vi "read_waveform.vi"(8 "error in (no error)":errorcluster, 10 "Small?":bool, 11 "Dust Event ID":i32) -> (0 "error out":errorcluster, 2 "multiplier":dbl, 3 "Waveform":T1)   [LabVIEW 2013]
uses:
  User Interface/Controls/Waveforms.ctl
  <vilib>/addons/h5labview/H5F_mode.ctl
  User Interface/Controls/Post_Signal.ctl
  User Interface/Controls/Role ID.ctl
  User Interface/Controls/Hardware ID.ctl
  <userlib>/_OpenG.lib/file/file.llb/File Exists - Scalar__ogtk.vi
  <vilib>/addons/h5labview/polymorph/H5A_read_var.vi
  <vilib>/addons/database/_DB Variant To Data/Database Variant To Data.xnode
  <vilib>/addons/h5labview/H5File.lvlib
  <vilib>/addons/h5labview/H5GroupObject.lvlib
  <vilib>/addons/h5labview/H5Attrib.lvlib
panel:
  out "Query Syntax":string
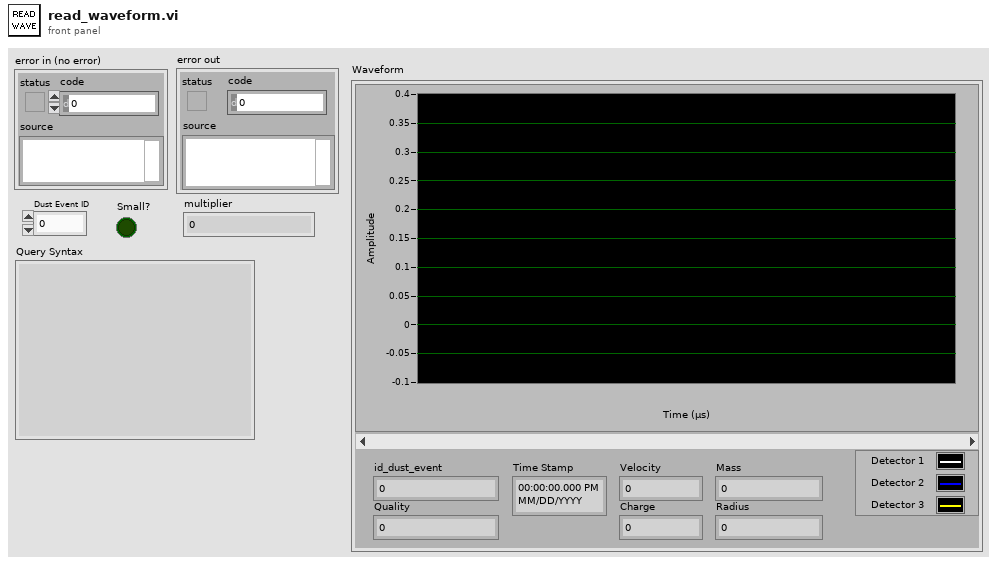
[diagram p1: front panel]
types:
  T1 = typedef "Waveforms.ctl" = cluster{"id_dust_event":u64, "Time Stamp":timestamp, "Velocity":dbl, "Mass":dbl, "Charge":dbl, "Radius":dbl, "Waveform Graph":sgl[][], "Quality":i32}
  T2 = typedef "H5File.lvlib/H5F_mode.ctl" = enum16{"read-only", "read-write", "overwrite", "create new", "open or create"}
  T3 = typedef "Role ID.ctl" = enum16{"First_Detector", "Second_Detector", "Third_Detector", "LeCroy_CH1", "LeCroy_CH2", "LeCroy_CH3", "LeCroy_CH4", "PSU", "DCS 1", "DCS 2"}
  T4 = typedef "Post_Signal.ctl" = cluster{"Integer Timestamp":i64, "Dust Event ID":i64, "Role ID":T3, "Data":sgl[], "Signal Length":i32, "dt":sgl, "Offset":dbl, "Hardware ID":T5}
  T5 = typedef "Hardware ID.ctl" = enum16{"Unknown", "CSA 1", "CSA 2", "CSA 3", "CSA 4", "CSA 5", "CSA 6", "DCS 1", "DCS 2"}
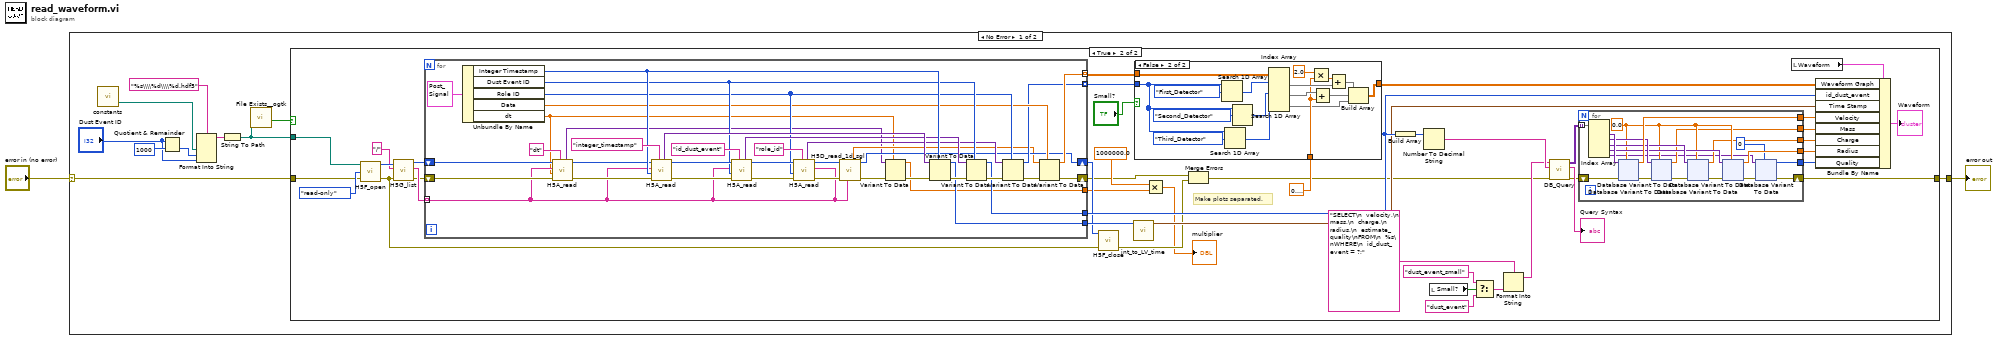
[diagram p0: block diagram]
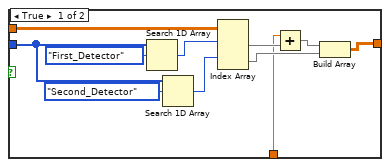
[diagram p3: hidden frame]
diagram:
  n1 = case shown="No Error" "error in (no error)" {
    selector: "error in (no error)" -> [w3 w302]
    tunnel: [w7 w302] -> w1
    frame No Error {
      n2 = call "constants.vi"() -> ("file path for Processed Signal .hdf5 files"=w4:path)  [unwired: 3 in, 2 out]
      n3 = Quotient & Remainder(x="Dust Event ID", y=1000) -> (floor(x/y)=w10:i32)  [unwired: 1 out]
      n4 = Format Into String(format string="%s\\\\%d\\\\%d.hdf5", w4, w10, "Dust Event ID") -> (resulting string=w8:string)  [unwired: 2 in, 1 out]
      n5 = String To Path(string=w8) -> (path=w5:path)
      n6 = call-poly <userlib>:"File Exists__ogtk.vi"("file path"=w5) -> ("exists"=w6:bool)  [unwired: 6 in, 1 out]
      n7 = case shown="True" w6 {
        tunnel: w5 -> [_ w56]
        tunnel: [w13 w54] -> w7
        tunnel: w3 -> [w13 w14]
        frame False {
        }
        frame True {
          # "Make plots separated."
          n8 = call <vilib>:"H5F_open.vi"("error in (no error)"=w14, "mode"=H5F_mode."read-only", "path"=w56) -> ("error out"=w20:errorcluster, "ref"=w53:i32)  [unwired: 1 in]
          n9 = call <vilib>:"H5G_list.vi"("error in (no error)"=w20, "group"="/", "ref"=w53) -> ("error out"=w25:errorcluster, "names"=w29:string[], "ref out"=w26:i32)  [unwired: 1 in, 1 out]
          n10 = for {
            shift-right: [w279] -> w17
            shift-left: w25 -> [w272]
            shift-right: [w278] -> w27
            shift-left: w26 -> [w274]
            tunnel: w29 -> [w265] mode=indexing
            tunnel: [w280] -> w31 mode=indexing
            tunnel: [w281] -> w32 mode=indexing
            tunnel: [w276] -> w50
            tunnel: [w277] -> w33
            tunnel: [w267] -> w15
            n11 = Unbundle By Name(T4 {"Integer Timestamp"=0, "Dust Event ID"=0, "Role ID"=enum."First_Detector", "Data"=[], "Signal Length"=0, "dt"=0.0, "Offset"=0.0, "Hardware ID"=enum."CSA 1"} ("Post_Signal 2")) -> ("Integer Timestamp"=w299:i64, "Dust Event ID"=w293:i64, "Role ID"=w287:T3, "Data"=w284:sgl[], "dt"=w264:sgl)
            n12 = call-poly <vilib>:"H5A_read.vi"("attrib_name"="dt", "error in (no error)"=w272, "default"=w264, "obj_name"=w265, "ref"=w274) -> ("error out"=w271:errorcluster, "ref out"=w273:i32, "value"=w268:variant)  [unwired: 2 in]
            n13 = call-poly <vilib>:"H5A_read.vi"("attrib_name"="integer_timestamp", "error in (no error)"=w271, "default"=w299, "obj_name"=w265, "ref"=w273) -> ("error out"=w295:errorcluster, "ref out"=w297:i32, "value"=w298:variant)  [unwired: 2 in]
            n14 = call-poly <vilib>:"H5A_read.vi"("attrib_name"="id_dust_event", "error in (no error)"=w295, "default"=w293, "obj_name"=w265, "ref"=w297) -> ("error out"=w291:errorcluster, "ref out"=w290:i32, "value"=w294:variant)  [unwired: 2 in]
            n15 = call-poly <vilib>:"H5A_read.vi"("attrib_name"="role_id", "error in (no error)"=w291, "default"=w287, "obj_name"=w265, "ref"=w290) -> ("error out"=w282:errorcluster, "ref out"=w283:i32, "value"=w288:variant)  [unwired: 2 in]
            n16 = call "H5D_read_1d_sgl.vi"("name"=w265, "error in (no error)"=w282, "ref"=w283) -> ("error out"=w270:errorcluster, "ref out"=w278:i32, "data"=w275:sgl[])  [unwired: 4 in]
            n17 = Variant To Data(error in=w270, type=w264, Variant=w268) -> (data=w267:sgl, error out=w269:errorcluster)
            n18 = Variant To Data(error in=w269, type=w299, Variant=w298) -> (data=w277:i64, error out=w292:errorcluster)
            n19 = Variant To Data(error in=w292, type=w293, Variant=w294) -> (data=w276:i64, error out=w286:errorcluster)
            n20 = Variant To Data(error in=w286, type=w287, Variant=w288) -> (data=w280:T3, error out=w285:errorcluster)
            n21 = Variant To Data(error in=w285, type=w284, Variant=w275) -> (data=w281:sgl[], error out=w279:errorcluster)
          }
          n22 = call <vilib>:"H5F_close.vi"("error in (no error)"=w20, "ref"=w27) -> ("error out"=w21:errorcluster)  [unwired: 3 in]
          n23 = call "int_to_LV_time.vi"("Integer Timestamp"=w33) -> ("time stamp"=w34:timestamp)  [unwired: 8 in, 1 out]
          n24 = case shown="False" "Small?" {
            tunnel: w31 -> [w243 w259]
            tunnel: w32 -> [w241 w256]
            tunnel: [w238 w251] -> w23
            tunnel: sgl 0.1 -> [w236 w248]
            frame True {
              n25 = Search 1D Array(1D array=w243, element=Role_ID."First_Detector") -> (index of element=w244:i32)  [unwired: 1 in]
              n26 = Search 1D Array(1D array=w243, element=Role_ID."Second_Detector") -> (index of element=w242:i32)  [unwired: 1 in]
              n27 = Index Array(array=w241, index (row) #1=w244, index (row) #2=w242) -> (element #1=w240:sgl[], element #2=w239:sgl[])  [unwired: 2 in]
              n28 = Add(x=w236, y=w240) -> (x+y=w237:sgl[])
              n29 = Build Array(w237, w239) -> (w238:sgl[][])
            }
            frame False {
              n30 = Search 1D Array(1D array=w259, element=Role_ID."First_Detector") -> (index of element=w261:i32)  [unwired: 1 in]
              n31 = Search 1D Array(1D array=w259, element=Role_ID."Third_Detector") -> (index of element=w257:i32)  [unwired: 1 in]
              n32 = Search 1D Array(1D array=w259, element=Role_ID."Second_Detector") -> (index of element=w258:i32)  [unwired: 1 in]
              n33 = Index Array(array=w256, index (row) #1=w261, index (row) #2=w258, index (row) #3=w257) -> (element #1=w255:sgl[], element #2=w254:sgl[], element #3=w247:sgl[])  [unwired: 3 in]
              n34 = Multiply(x=sgl 2.0, y=w248) -> (x*y=w250:sgl)
              n35 = Add(x=w254, y=w248) -> (x+y=w252:sgl[])
              n36 = Add(x=w250, y=w255) -> (x+y=w253:sgl[])
              n37 = Build Array(w253, w252, w247) -> (w251:sgl[][])
            }
          }
          n38 = Multiply(x=1000000.0, y=w15) -> (x*y=→"multiplier":dbl)
          n39 = Merge Errors(w17, w21) -> (w19:errorcluster)
          n40 = Build Array(w50) -> (w51:i64[])
          n41 = Number To Decimal String(number=w51) -> (decimal integer string=w52:string[])  [unwired: 1 in]
          n42 = local read "Small?"() -> (w38:bool)
          n43 = Select(t="dust_event_small" ("resulting string"), s=w38, f="dust_event" ("resulting string")) -> (s? t:f=w37:string)
          n44 = Format Into String(format string="SELECT\n  velocity,\n  mass,\n  charge,\n  radius,\n  estimate_quality\nFROM\n  %s\nWHERE\n  id_dust_event = ?;" ("SQL query"), w37) -> (resulting string=w49:string)  [unwired: 2 in, 1 out]
          n45 = call "DB_Query.vi"("error in (no error)"=w19, "Parameters"=w52, "Parameterized Query"=w49) -> ("error out"=w46:errorcluster, "Query in Standard Format"=→"Query Syntax":string, "Results"=w47:variant[][])  [unwired: 6 in]
          n46 = for {
            tunnel: w47 -> [w74] mode=indexing
            shift-right: [w60] -> w54
            shift-left: w46 -> [w75]
            tunnel: [w71] -> w41
            tunnel: [w64] -> w42
            tunnel: [w63] -> w43
            tunnel: [w62] -> w44
            tunnel: [w57] -> w45
            w65 = 0.0 ("Velocity")
            n47 = Index Array(array=w74) -> (element #1=w73:variant, element #2=w70:variant, element #3=w68:variant, element #4=w66:variant, element #5=w59:variant)  [unwired: 5 in]
            n48 = xnode "Database Variant To Data"("database variant"=w73, "error in (no error)"=w75, "type"=w65) -> ("data"=w71:dbl, "error out"=w72:errorcluster)
            n49 = xnode "Database Variant To Data"("database variant"=w70, "error in (no error)"=w72, "type"=w65) -> ("data"=w64:dbl, "error out"=w69:errorcluster)
            n50 = xnode "Database Variant To Data"("database variant"=w68, "error in (no error)"=w69, "type"=w65) -> ("data"=w63:dbl, "error out"=w67:errorcluster)
            n51 = xnode "Database Variant To Data"("database variant"=w66, "error in (no error)"=w67, "type"=w65) -> ("data"=w62:dbl, "error out"=w61:errorcluster)
            n52 = xnode "Database Variant To Data"("database variant"=w59, "error in (no error)"=w61, "type"=i64 0 ("Dust Event ID")) -> ("data"=w57:i64, "error out"=w60:errorcluster)
          }
          n53 = local read "Waveform"() -> (w30:T1)
          n54 = Bundle By Name(cluster=w30, "Waveform Graph"=w23, "id_dust_event"=w50, "Time Stamp"=w34, "Velocity"=w41, "Mass"=w42, "Charge"=w43, "Radius"=w44, "Quality"=w45) -> (→"Waveform":T1)
        }
      }
    }
    frame Error {
    }
  }
  "error out" <- w1
